vi "Rotation3d_Create_AxisAngle.vi"(9 "Angle":dbl, 11 "Axis Vector":dbl[](array[numeric])=[0.0, 0.0, 0.0]) -> (3 "Rotation3d":T1={"Q_quaternion"={"R"=1.0, "V"=[0.0, 0.0, 0.0]}})   [LabVIEW 2019, in "Trajectory_Library.lvlib"]
doc: "Constructs a Rotation2d with the given radian value. The x and y don't have to be normalized.\n\nParmeters:\n - value - The value of the angle in radians.\n\nReturns\n - rotation data structure"
uses:
  ROTATION3D.ctl
  QUATERNION.ctl
  Trajectory_Library.lvlib
  <vilib>/Analysis/Matrix/NI_Matrix.lvlib
  <vilib>/Analysis/Matrix/Numeric/Conversions/Array To Matrix - RA.vi
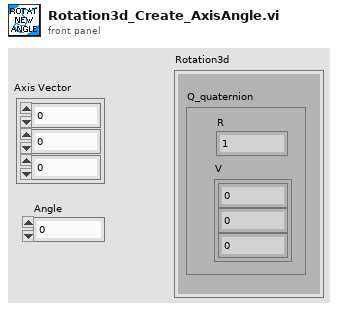
[diagram p1: front panel]
types:
  T1 = typedef "Trajectory_Library.lvlib/ROTATION3D.ctl" = cluster{"Q_quaternion":T2}
  T2 = typedef "Trajectory_Library.lvlib/QUATERNION.ctl" = cluster{"R":dbl, "V":dbl[]}
  T3 = typedef "NI_Matrix.lvlib/RealMatrix.ctl" = dbl[][]
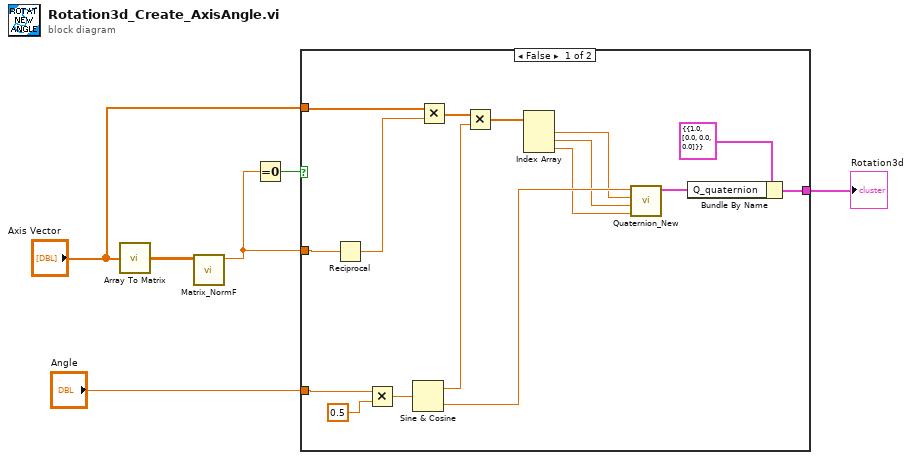
[diagram p0: block diagram]
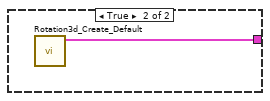
[diagram p2: hidden frame]
diagram:
  n1 = call-poly <vilib>:"Array To Matrix.vi"("Real 1D Array"="Axis Vector") -> ("Real Matrix (Column Vector)"=w6:T3)
  n2 = call "Matrix_NormF.vi"("input matrix"=w6) -> ("normF"=w3:dbl)  [unwired: 9 in, 1 out]
  n3 = Equal To 0?(x=w3) -> (x = 0?=w5:bool)
  n4 = case shown="False" w5 {
    tunnel: [w20 w23] -> w4
    tunnel: w3 -> [w13 _]
    tunnel: "Axis Vector" -> [w14 _]
    tunnel: "Angle" -> [w12 _]
    frame False {
      n5 = Reciprocal(x=w13) -> (1/x=w19:dbl)
      n6 = Multiply(x=w12, y=0.5) -> (x*y=w17:dbl)
      n7 = Sine & Cosine(0:w17) -> (1:w15:dbl, 2:w11:dbl)
      n8 = Multiply(x=w14, y=w19) -> (x*y=w16:dbl[])
      n9 = Multiply(x=w16, y=w15) -> (x*y=w10:dbl[])
      n10 = Index Array(array=w10) -> (element #1=w9:dbl, element #2=w8:dbl, element #3=w7:dbl)  [unwired: 3 in]
      n11 = call "Quaternion_New.vi"("Z"=w7, "Y"=w8, "X"=w9, "W"=w11) -> ("out Quaternion"=w22:T2)  [unwired: 7 in]
      n12 = Bundle By Name(cluster=T1 {"Q_quaternion"={"R"=1.0, "V"=[0.0, 0.0, 0.0]}} ("ROTATION3D"), "Q_quaternion"=w22) -> (w20:T1)
    }
    frame True {
      n13 = call "Rotation3d_Create_Default.vi"() -> ("ROTATION3D"=w23:T1)  [unwired: 11 in]
    }
  }
  "Rotation3d" <- w4
